vi "String Indicator.vi"(10 "String Indicator":string, 11 "String Indicator in":refnum<class "String Indicator.lvclass">) -> (3 "String Indicator out":refnum<class "String Indicator.lvclass">)   [LabVIEW 2021, in "String Indicator Event.lvlib" / "String Indicator.lvclass"]
uses:
  String Indicator.lvclass
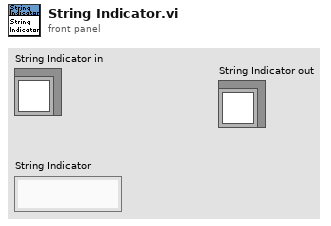
[diagram p1: front panel]
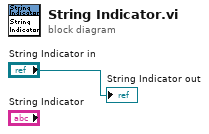
[diagram p0: block diagram]
diagram:
  "String Indicator out" <- "String Indicator in"
